vi "Read Recorded File.vi"(11 "Filename":string) -> (2 "Turn":dbl[](array[numeric]), 3 "Speed":dbl[](array[numeric]))   [LabVIEW 2019]
uses:
  <vilib>/Utility/file.llb/Read Delimited Spreadsheet (DBL).vi
panel:
  out "array w/ subset deleted":dbl[][](array[numeric])
  out "all rows":dbl[][](array[numeric])
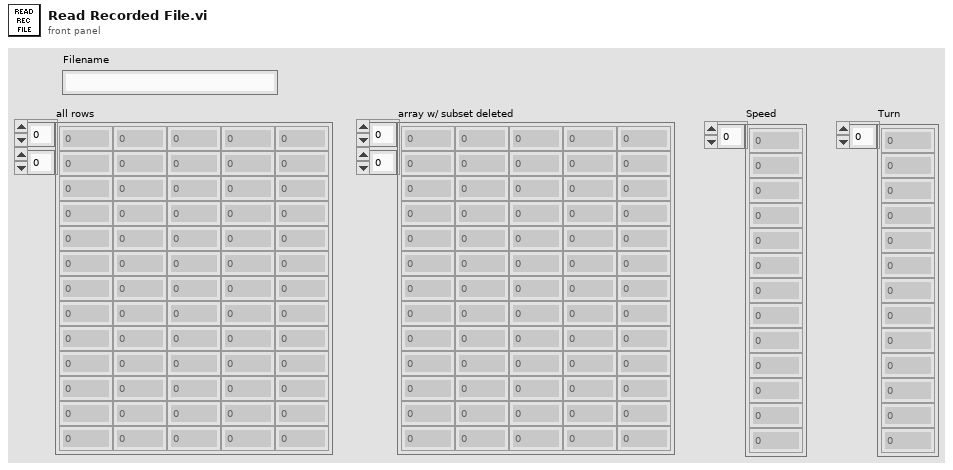
[diagram p1: front panel]
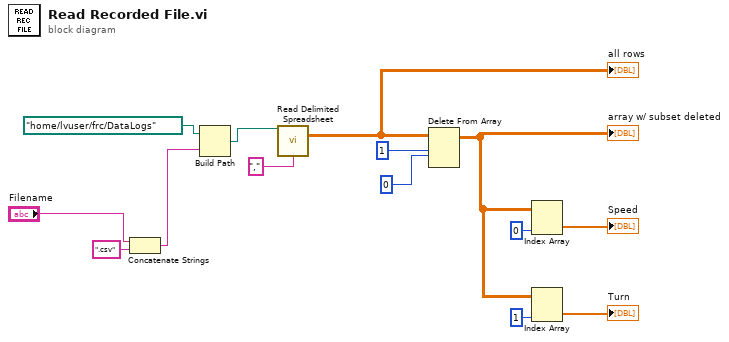
[diagram p0: block diagram]
diagram:
  n1 = Concatenate Strings("Filename", ".csv" ("string")) -> (w2:string)
  n2 = Build Path(base path=path "/home/lvuser/frc/DataLogs", name or relative path=w2) -> (appended path=w4:path)
  n3 = call-poly <vilib>:"Read Delimited Spreadsheet.vi"("file path (dialog if empty)"=w4, "delimiter (\\t)"="," ("delimiter (\\t)")) -> ("all rows"=w9:dbl[][])  [unwired: 8 in, 5 out]
  "all rows" <- w9
  n4 = Delete From Array(array=w9, length=1, index (row)=0) -> (array with subset deleted=w14:dbl[][])  [unwired: 1 in, 1 out]
  "array w/ subset deleted" <- w14
  n5 = Index Array(array=w14, index (col)=0 ("disabled index (col)")) -> (element=→"Speed":dbl[])  [unwired: 1 in]
  n6 = Index Array(array=w14, index (col)=1 ("disabled index (col)")) -> (element=→"Turn":dbl[])  [unwired: 1 in]
